vi "jsonPath.vi"(8 "error in (no error)":errorcluster, 11 "json path in":string="$.home.room.table.lamp") -> (0 "error out":errorcluster, 3 "output array of keys":string[](array[string]))   [LabVIEW 2015, in "Zen Analytics.lvclass"]
uses:
  Zen Analytics.lvclass
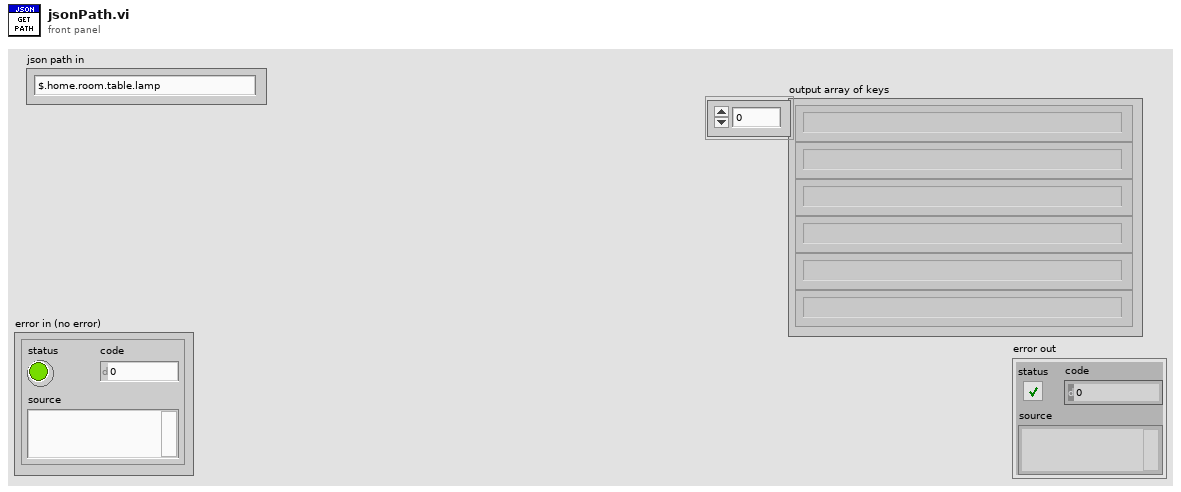
[diagram p1: front panel]
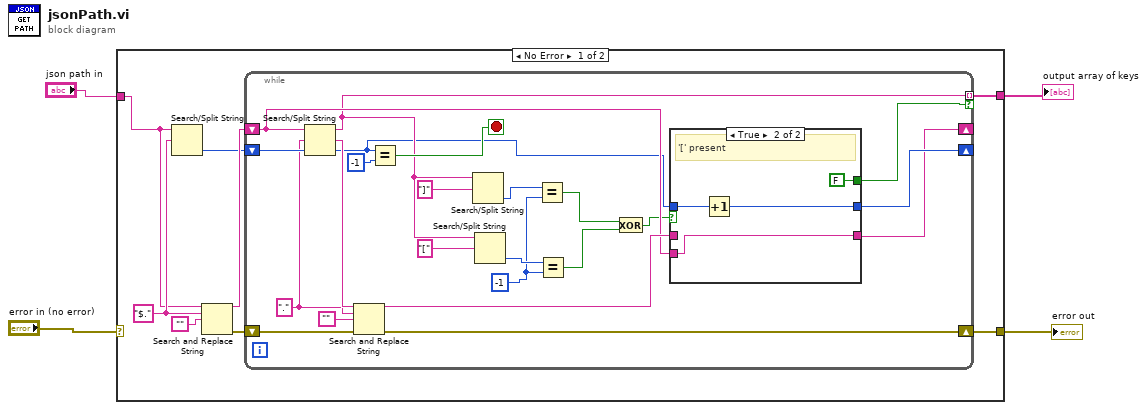
[diagram p0: block diagram]
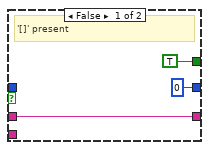
[diagram p2: hidden frame]
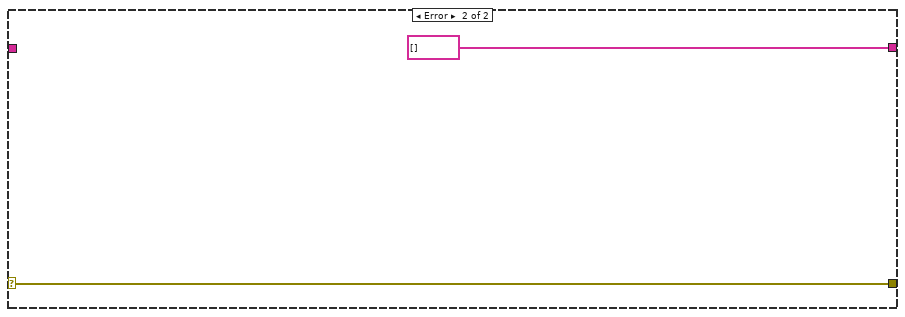
[diagram p3: hidden frame]
diagram:
  n1 = case shown="No Error" "error in (no error)" {
    selector: "error in (no error)" -> [_ w43]
    tunnel: "json path in" -> [w9 _]
    tunnel: [w6 w43] -> w2
    tunnel: [w7 string[] []] -> w1
    frame No Error {
      w12 = "$." ("search string/char (-)")
      n2 = Search/Split String(string=w9, search string/char (-)=w12) -> (offset of match=w5:i32)  [unwired: 1 in, 2 out]
      n3 = Search and Replace String(input string=w9, search string=w12, replace string="") -> (result string=w10:string, error out=w8:errorcluster)  [unwired: 5 in, 2 out]
      n4 = while {
        shift-right: [w24] -> _
        shift-left: w10 -> [w22]
        tunnel: [w21] -> w7 mode=indexing if=w15
        shift-right: [w31] -> w6
        shift-left: w8 -> [w32]
        shift-right: [w27] -> _
        shift-left: w5 -> [w26]
        stop <- w30 stop-if-true
        w18 = -1 ("y")
        w23 = "." ("search string/char (-)")
        n5 = Search/Split String(string=w22, search string/char (-)=w23, offset (0)=w26) -> (substring before match=w21:string, match + rest of string=w33:string, offset of match=w16:i32)
        n6 = Search and Replace String(input string=w33, search string=w23, replace string="", error in=w32) -> (result string=w25:string, error out=w31:errorcluster)  [unwired: 4 in, 2 out]
        n7 = Equal?(x=w16, y=-1) -> (x = y?=w30:bool)
        n8 = Search/Split String(string=w21, search string/char (-)="]") -> (offset of match=w19:i32)  [unwired: 1 in, 2 out]
        n9 = Search/Split String(string=w21, search string/char (-)="[") -> (offset of match=w28:i32)  [unwired: 1 in, 2 out]
        n10 = Equal?(x=w19, y=w18) -> (x = y?=w14:bool)
        n11 = Equal?(x=w28, y=w18) -> (x = y?=w13:bool)
        n12 = Exclusive Or(1:w13, 2:w14) -> (0:w17:bool)
        n13 = case shown="True" w17 {
          tunnel: w16 -> [_ w41]
          tunnel: [0 w40] -> w27
          tunnel: w25 -> [w37 _]
          tunnel: [w37 w42] -> w24
          tunnel: w22 -> [_ w42]
          tunnel: [TRUE FALSE] -> w15
          frame False {
            # "'[]' present"
          }
          frame True {
            # "'[' present"
            n14 = Increment(x=w41) -> (x+1=w40:i32)
          }
        }
      }
    }
    frame Error {
    }
  }
  "output array of keys" <- w1
  "error out" <- w2
